vi "Get Active BuildSpec.vi"(11 "Project Sync Tools in":refnum<class "Project Sync Tools.lvclass">) -> (2 "Build Spec Parameters":T1, 3 "Project Sync Tools out":refnum<class "Project Sync Tools.lvclass">)   [LabVIEW 2019, in "Project Sync Tools.lvclass"]
uses:
  Project Sync Tools.lvclass
  TypeDefs/BuildSpec Raw Parameters.ctl
  Project Sync Tools.lvclass/Project Sync Tools.ctl
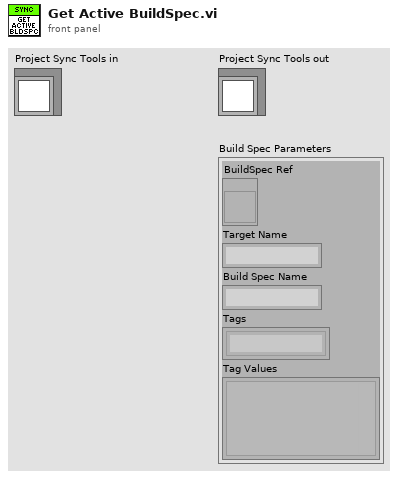
[diagram p1: front panel]
types:
  T1 = typedef "Project Sync Tools.lvclass/BuildSpec Raw Parameters.ctl" = cluster{"BuildSpec Ref":refnum<vi>, "Target Name":string, "Build Spec Name":string, "Tags":string[], "Tag Values":variant[]}
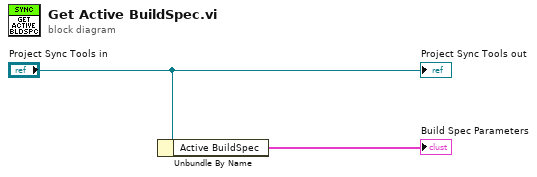
[diagram p0: block diagram]
diagram:
  n1 = Unbundle By Name("Project Sync Tools in") -> ("Active BuildSpec"=→"Build Spec Parameters":T1)
  "Project Sync Tools out" <- "Project Sync Tools in"
